vi "Untitled 1.vi"() -> ()   [LabVIEW 2016]
panel:
  out "s4":string
  in  "s1":string
  in  "Stop Button":bool
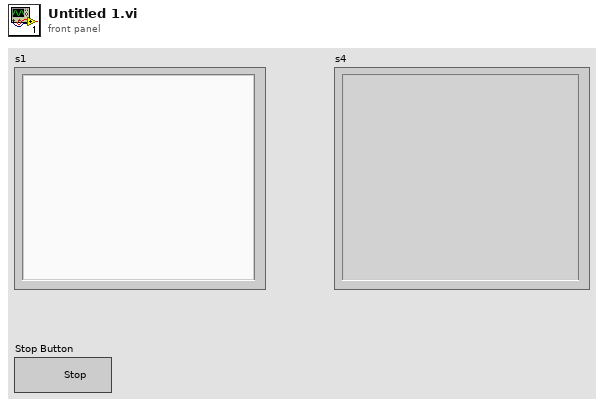
[diagram p1: front panel]
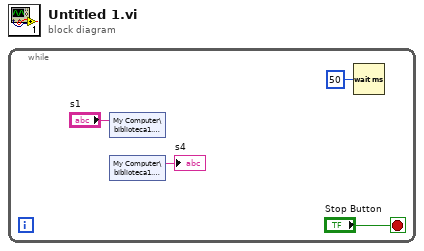
[diagram p0: block diagram]
diagram:
  n1 = while {
    stop <- "Stop Button" stop-if-true
    n2 = shared-variable "My Computer\\biblioteca1.lvlib\\s1"("s1") -> ()  [unwired: 1 in, 1 out]
    n3 = shared-variable "My Computer\\biblioteca1.lvlib\\s4"() -> (→"s4":string)  [unwired: 1 in, 1 out]
    n4 = Wait (ms)(milliseconds to wait=u32 50) -> ()  [unwired: 1 out]
  }
